vi "MAIN_init_ramp_autofocus.vi"(3 "error in":errorcluster, 4 "Total range (nm)":u32=2000, 5 "z step (nm)":u32=50, 6 "queue piezo":refnum<queue>) -> (0 "error out":errorcluster, 1 "Ramp":dbl[](array[numeric]), 2 "z0":dbl)   [LabVIEW 2015]
uses:
  CONTROLS/Q_MCL_piezo_element.ctl
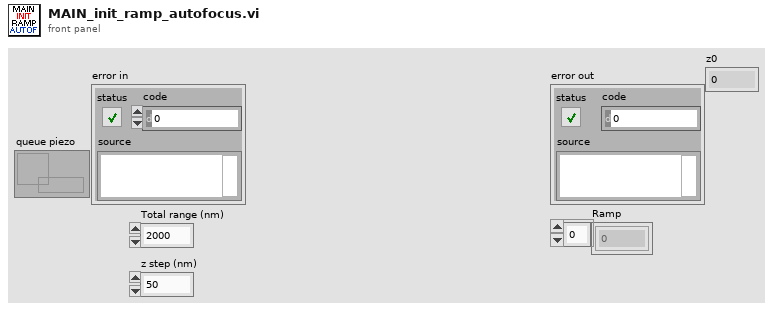
[diagram p1: front panel]
types:
  T1 = typedef "Q_MCL_piezo_element.ctl" = cluster{"variant":variant, "Instruction":enum16{"Piezo_idle", "Piezo_initialize", "Piezo_error", "Piezo_security_stop", "Piezo_read_z", "Piezo_move_z", "Piezo_keyboard_move", "Piezo_close_autofocus_calibration_ramp", "Piezo_change_init_state", "Piezo_init_autofocus", "Piezo_init_autofocus_merFISH_TL", "Piezo_autofocus", "Piezo_autofocus_merFISH_TL", "Piezo_stop_autofocus", "Piezo_stop_autofocus_merFISH_TL", "Piezo_autofocus_lost", "Piezo_resume_autofocus_merFISH_TL", "Piezo_check_z_position_merFISH_TL", "Piezo_init_ramp", "Piezo_move_z_ramp", "Piezo_close_ramp", "Piezo_close_merFISH", "Piezo_stop"}}
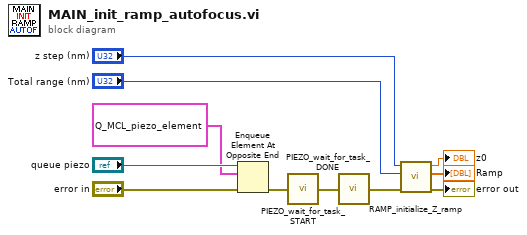
[diagram p0: block diagram]
diagram:
  n1 = Enqueue Element At Opposite End(queue="queue piezo", element=T1 {"variant"=variant, "Instruction"=enum."Piezo_init_ramp"}, error in (no error)="error in") -> (error out=w9:errorcluster)  [unwired: 1 in, 2 out]
  n2 = call "PIEZO_wait_for_task_START.vi"("error in"=w9) -> ("error out"=w8:errorcluster)
  n3 = call "PIEZO_wait_for_task_DONE.vi"("error in"=w8) -> ("error out"=w6:errorcluster)
  n4 = call "RAMP_initialize_Z_ramp.vi"("error in"=w6, "Total range (nm)"="Total range (nm)", "dZ (nm)"="z step (nm)") -> ("error out"=→"error out":errorcluster, "Ramp"=→"Ramp":dbl[], "z0"=→"z0":dbl)  [unwired: 2 in, 1 out]
